vi "Atoi, four hex scalars.vi"(5 "default (0)":i32, 6 "offset (0)":i32, 7 "string 4":string, 8 "string 3":string, 9 "string 2":string, 10 "string 1":string) -> (0 "number 4":i32 format="%.0x", 1 "number 3":i32 format="%.0x", 2 "number 2":i32 format="%.0x", 3 "number 1":i32 format="%.0x")   [LabVIEW 2010]
doc: "This function converts four strings to four signed hexadecimal integers (without rounding)."
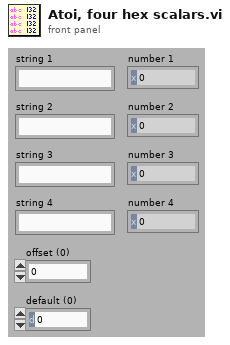
[diagram p1: front panel]
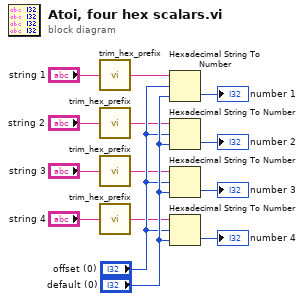
[diagram p0: block diagram]
diagram:
  n1 = call "trim_hex_prefix.vi"("string in"="string 1") -> ("string out"=w7:string)
  n2 = call "trim_hex_prefix.vi"("string in"="string 2") -> ("string out"=w1:string)
  n3 = call "trim_hex_prefix.vi"("string in"="string 3") -> ("string out"=w3:string)
  n4 = call "trim_hex_prefix.vi"("string in"="string 4") -> ("string out"=w5:string)
  n5 = Hexadecimal String To Number(string=w7, offset="offset (0)", default (0uL)="default (0)") -> (number=→"number 1":i32)  [unwired: 1 out]
  n6 = Hexadecimal String To Number(string=w1, offset="offset (0)", default (0uL)="default (0)") -> (number=→"number 2":i32)  [unwired: 1 out]
  n7 = Hexadecimal String To Number(string=w3, offset="offset (0)", default (0uL)="default (0)") -> (number=→"number 3":i32)  [unwired: 1 out]
  n8 = Hexadecimal String To Number(string=w5, offset="offset (0)", default (0uL)="default (0)") -> (number=→"number 4":i32)  [unwired: 1 out]
